vi "Periodic Tasks.vi"(8 "error in":errorcluster) -> ()   [LabVIEW 2017]
doc: "This VI runs in parallel to other tasks. It can contain as many user-defined periodic loops as you need. These can carry out PID or other sorts of timed response."
uses:
  <vilib>/Rock Robotics/Network Tables/NT Write Numeric Array.vi
  <vilib>/Rock Robotics/Network Tables/NT Write Boolean Array.vi
  Robot Global Data.vi
  <vilib>/Rock Robotics/WPI/ThirdParty/CanMotor/TalonSRX/WPI_CANTalonSRX_APIControlMode.ctl
  <vilib>/Rock Robotics/Network Tables/NT Read Number.vi
  <vilib>/Rock Robotics/Network Tables/NT Write Boolean.vi
panel:
  in  "corrector":dbl=-0.5
  in  "Slow Range":dbl=45.0
  out "Speed Closed Loop Plots 2":cluster{dbl, "Sensor Velocity":dbl}(graph)
  in  "Motor Power In":dbl=1.0
  in  "Target Range":dbl=0.5
  in  "Min Power":dbl=0.17
  out "Speed Closed Loop Plots":cluster{dbl, "Sensor Velocity":dbl}(graph)
  out "RightEncoder":dbl
  out "LeftEncoder":dbl
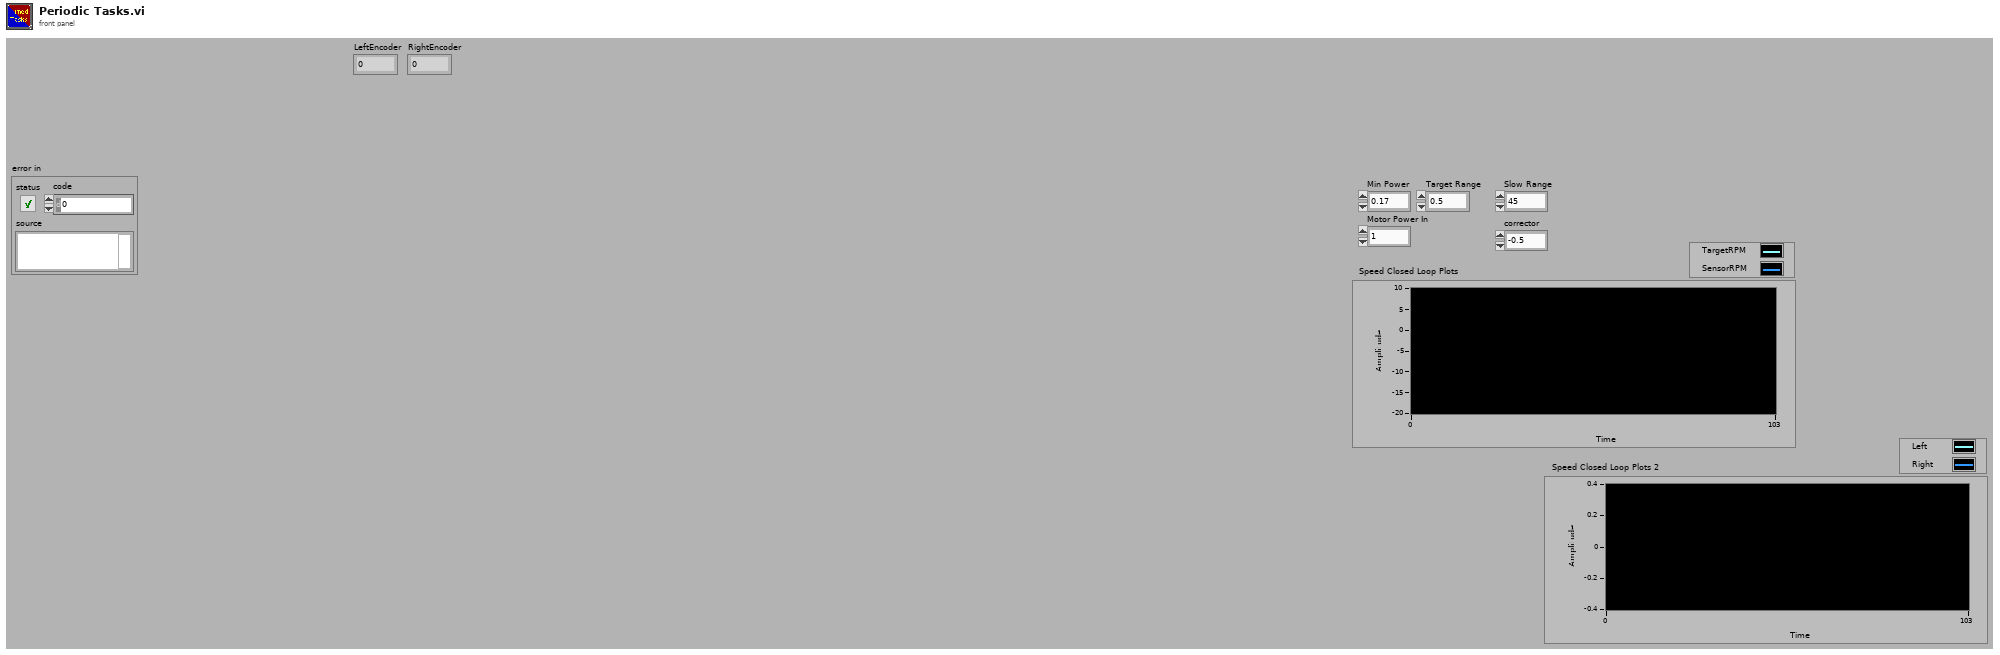
[diagram p1: front panel]
types:
  T1 = typedef "WPI_JoystickDevRef.ctl" = cluster{"Device":T2}
  T2 = typedef "WPI_JoystickDeviceEnum.ctl" = enum16{"USB 0", "USB 1", "USB 2", "USB 3", "USB 4", "USB 5"}
  T3 = cluster{"Yaw":dbl, "Roll":dbl, "Pitch":dbl, "Heading":dbl, "Fused Heading":dbl}
  T4 = typedef "WPI_CompressorDevRef.ctl" = cluster{"DevStatus":errorcluster, "Pneumatics Control Module":u8}
  T5 = enum16{"Integer", "Float", "Boolean", "Enum", "String"}
  T6 = typedef "WPI_CANTalonSRX_APIControlMode.ctl" = enum8{"Percent VBus", "Speed", "Position", "Slave", "Unchanged / Invalid", "Voltage Compensation", "Current", "Motion Profile", "Motion Magic"}
  T7 = typedef "WPI_DriverStationRobotMode2.ctl" = enum16{"Autonomous Disabled", "Autonomous Enabled", "Teleop Disabled", "Teleop Enabled", "Disconnected", "Finish", "Test Disabled", "Test Enabled", "Emergency Stopped"}
  T8 = cluster{"Buttons[0]":bool, "Buttons[1]":bool, "Buttons[2]":bool, "Buttons[3]":bool, "Buttons[4]":bool, "Buttons[5]":bool, "Buttons[6]":bool, "Buttons[7]":bool, "Buttons[8]":bool, "Buttons[9]":bool, "Buttons[10]":bool, "Buttons[11]":bool}
  T9 = cluster{"Left Motor Power":dbl, "Right Motor Power":dbl}
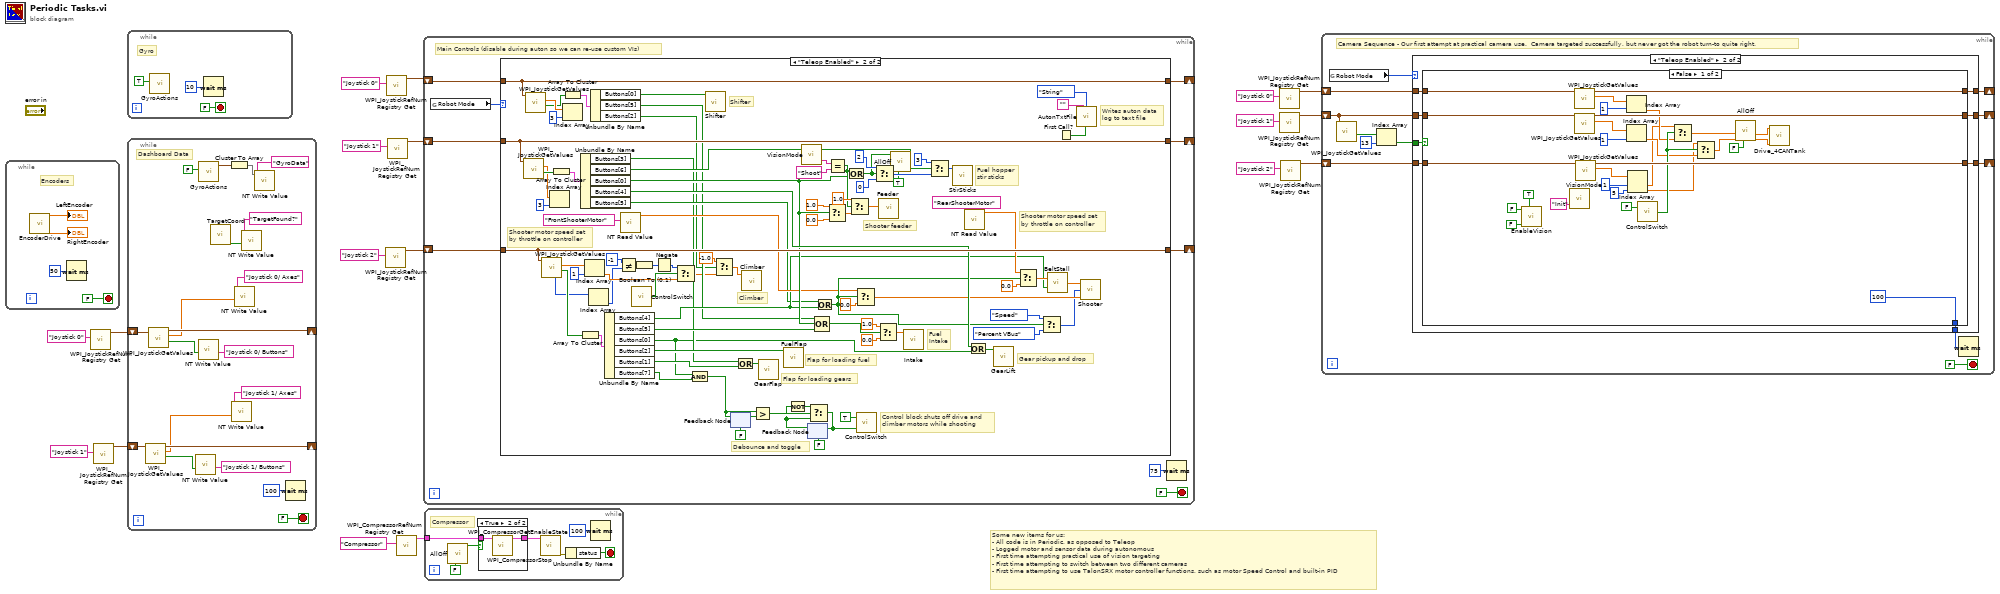
[diagram p0: block diagram]
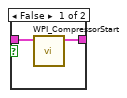
[diagram p2: hidden frame]
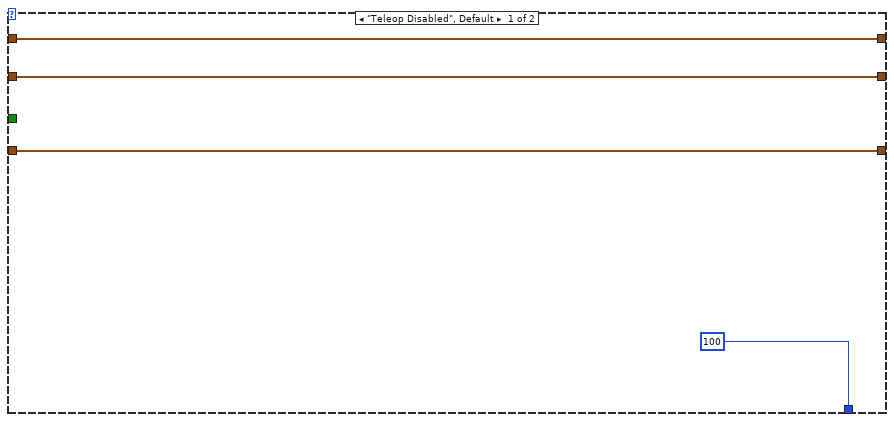
[diagram p3: hidden frame]
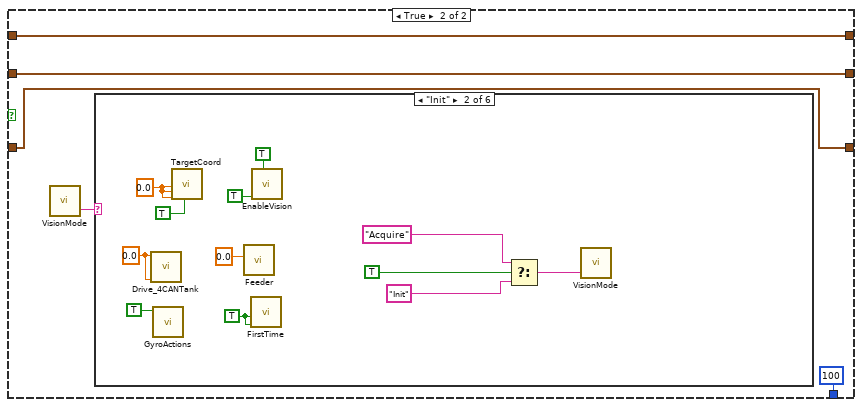
[diagram p4: hidden frame]
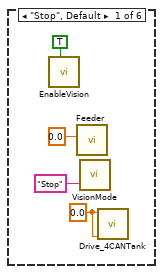
[diagram p5: hidden frame]
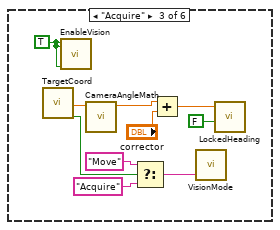
[diagram p6: hidden frame]
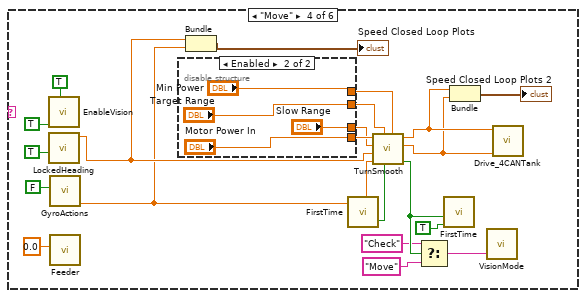
[diagram p7: hidden frame]
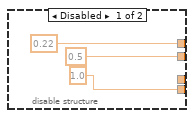
[diagram p8: hidden frame]
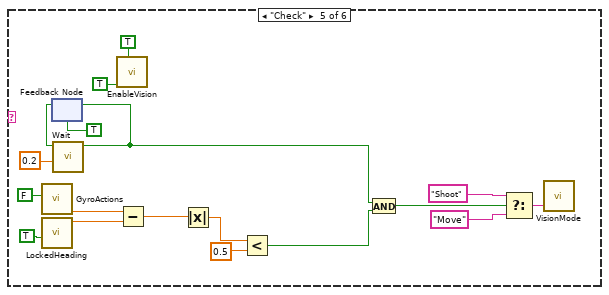
[diagram p9: hidden frame]
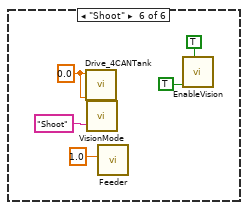
[diagram p10: hidden frame]
diagram:
  # "Some new items for us:\n- All code is in Periodic, as opposed to Teleop\n- Logged motor and sensor data during autonomous\n- First time attempting practical use of vision targeting\n- First time attempting to switch between two different cameras\n- First time attempting to use TalonSRX motor controller functions, such as motor Speed Control and built-in PID"
  n1 = while {
    stop <- FALSE stop-if-true
    # "Encoders"
    n2 = call "EncoderDrive.vi"() -> ("RightEncder"=→"RightEncoder":dbl, "LeftEncoder"=→"LeftEncoder":dbl)  [unwired: 10 in]
    n3 = Wait (ms)(milliseconds to wait=u32 50) -> ()  [unwired: 1 out]
  }
  n4 = call <vilib>:"WPI_JoystickRefNum Registry Get.vi"("refnum name"="Joystick 0") -> ("JoystickDevRef"=w16:T1)  [unwired: 9 in, 1 out]
  n5 = call <vilib>:"WPI_JoystickRefNum Registry Get.vi"("refnum name"="Joystick 1") -> ("JoystickDevRef"=w15:T1)  [unwired: 9 in, 1 out]
  n6 = while {
    stop <- FALSE stop-if-true
    # "Gyro"
    n7 = call "GyroActions.vi"("Update?"=TRUE) -> ()  [unwired: 9 in, 2 out]
    n8 = Wait (ms)(milliseconds to wait=u32 10) -> ()  [unwired: 1 out]
  }
  n9 = while {
    shift-right: [w41] -> _
    shift-left: w16 -> [w42]
    shift-right: [w33] -> _
    shift-left: w15 -> [w34]
    stop <- FALSE stop-if-true
    # "Dashboard Data"
    n10 = call <vilib>:"WPI_JoystickGetValues.vi"("JoystickDevRef"=w34) -> ("Buttons"=w37:bool[], "Axes"=w32:dbl[], "JoystickDevRef"=w33:T1)  [unwired: 6 in, 2 out]
    n11 = call <vilib>:"WPI_JoystickGetValues.vi"("JoystickDevRef"=w42) -> ("Buttons"=w39:bool[], "Axes"=w38:dbl[], "JoystickDevRef"=w41:T1)  [unwired: 6 in, 2 out]
    n12 = call-poly <vilib>:"NT Write Value.vi"("Boolean Array"=w37, "Name"="Joystick 1/ Buttons") -> ()  [unwired: 9 in, 1 out]
    n13 = call-poly <vilib>:"NT Write Value.vi"("Boolean Array"=w39, "Name"="Joystick 0/ Buttons") -> ()  [unwired: 9 in, 1 out]
    n14 = call "GyroActions.vi"("Update?"=FALSE) -> ("YRPHfH"=w29:T3)  [unwired: 9 in, 1 out]
    n15 = call "TargetCoord.vi"() -> ("Target?"=w27:bool)  [unwired: 17 in, 2 out]
    n16 = Cluster To Array(cluster=w29) -> (array=w45:dbl[])
    n17 = call-poly <vilib>:"NT Write Value.vi"("Numeric Array"=w32, "Name"="Joystick 1/ Axes") -> ()  [unwired: 9 in, 1 out]
    n18 = call-poly <vilib>:"NT Write Value.vi"("Numeric Array"=w38, "Name"="Joystick 0/ Axes") -> ()  [unwired: 9 in, 1 out]
    n19 = call-poly <vilib>:"NT Write Value.vi"("Boolean"=w27, "Name"="TargetFound?") -> ()  [unwired: 9 in, 1 out]
    n20 = call-poly <vilib>:"NT Write Value.vi"("Numeric Array"=w45, "Name"="GyroData") -> ()  [unwired: 9 in, 1 out]
    n21 = Wait (ms)(milliseconds to wait=u32 100) -> ()  [unwired: 1 out]
  }
  n22 = call <vilib>:"WPI_JoystickRefNum Registry Get.vi"("refnum name"="Joystick 2") -> ("JoystickDevRef"=w9:T1)  [unwired: 9 in, 1 out]
  n23 = call <vilib>:"WPI_JoystickRefNum Registry Get.vi"("refnum name"="Joystick 0") -> ("JoystickDevRef"=w11:T1)  [unwired: 9 in, 1 out]
  n24 = call <vilib>:"WPI_JoystickRefNum Registry Get.vi"("refnum name"="Joystick 1") -> ("JoystickDevRef"=w10:T1)  [unwired: 9 in, 1 out]
  n25 = call <vilib>:"WPI_CompressorRefNum Registry Get.vi"("refnum name"="Compressor") -> ("CompressorDevRef"=w3:T4)  [unwired: 9 in, 1 out]
  n26 = while {
    shift-right: [w47] -> _
    shift-left: w11 -> [w52]
    shift-right: [w48] -> _
    shift-left: w10 -> [w51]
    shift-right: [w49] -> _
    shift-left: w9 -> [w50]
    stop <- FALSE stop-if-true
    # "Main Controls (disable during auton so we can re-use custom VIs)"
    n27 = global read "Robot Global Data.vi" "Robot Mode"() -> (w46:T7)
    n28 = case shown="\"Teleop Enabled\"" w46 {
      tunnel: w52 -> [w57 w121]
      tunnel: w51 -> [w56 w134]
      tunnel: w50 -> [w55 w135]
      tunnel: [w55 w135] -> w49
      tunnel: [w56 w134] -> w48
      tunnel: [w57 w121] -> w47
      frame "Teleop Disabled", Default {
      }
      frame "Teleop Enabled" {
        # "Shifter"
        # "Climber"
        # "Control block shuts off drive and\nclimber motors while shooting"
        # "Shooter motor speed set\nby throttle on controller"
        # "Fuel hopper\nstir sticks"
        # "Shooter feeder"
        # "Fuel\nIntake"
        # "Gear pickup and drop"
        # "Flap for loading gears"
        # "Flap for loading fuel"
        # "Shooter motor speed set\nby throttle on controller"
        # "Debounce and toggle"
        # "Writes auton data\nlog to text file"
        n29 = call <vilib>:"WPI_JoystickGetValues.vi"("JoystickDevRef"=w134) -> ("Buttons"=w132:bool[], "Axes"=w123:dbl[])  [unwired: 6 in, 3 out]
        n30 = call <vilib>:"WPI_JoystickGetValues.vi"("JoystickDevRef"=w121) -> ("Buttons"=w114:bool[], "Axes"=w119:dbl[])  [unwired: 6 in, 3 out]
        n31 = call <vilib>:"WPI_JoystickGetValues.vi"("JoystickDevRef"=w135) -> ("Buttons"=w140:bool[], "Axes"=w143:dbl[], "POVs"=w67:i16[])  [unwired: 6 in, 2 out]
        n32 = Index Array(array=w123, index=3) -> ()  [unwired: 1 out]
        n33 = Array To Cluster(array=w132) -> (cluster=w133:T8)
        n34 = Array To Cluster(array=w114) -> (cluster=w115:T8)
        n35 = Index Array(array=w119, index=3) -> ()  [unwired: 1 out]
        n36 = Array To Cluster(array=w140) -> (cluster=w141:T8)
        n37 = Unbundle By Name(w133) -> ("Buttons[3]"=w79:bool, "Buttons[6]"=w85:bool, "Buttons[0]"=w107:bool, "Buttons[4]"=w124:bool, "Buttons[5]"=w86:bool)
        n38 = Index Array(array=w143, index=1) -> (element=w64:dbl)
        n39 = Index Array(array=w67) -> (element=w63:i16)  [unwired: 1 in]
        n40 = Unbundle By Name(w115) -> ("Buttons[0]"=w113:bool, "Buttons[5]"=w84:bool, "Buttons[2]"=w82:bool)
        n41 = Unbundle By Name(w141) -> ("Buttons[4]"=w87:bool, "Buttons[5]"=w97:bool, "Buttons[0]"=w60:bool, "Buttons[2]"=w136:bool, "Buttons[1]"=w77:bool, "Buttons[7]"=w78:bool)
        n42 = Not Equal?(x=i16 -1, y=w63) -> (x != y?=w61:bool)
        n43 = call-poly <vilib>:"NT Read Value.vi"("Name"="FrontShooterMotor") -> ("Numeric"=w93:dbl)  [unwired: 9 in, 1 out]
        n44 = call "ControlSwitch.vi"() -> ("ControlsSwitchOut"=w65:bool)  [unwired: 2 in]
        n45 = Boolean To (0,1)(Boolean=w61) -> (0, 1=w59:i16)
        n46 = Negate(x=w59) -> (-x=w58:i16)
        n47 = Select(t=w58, s=w65, f=w64) -> (s? t:f=w66:dbl)
        n48 = And(x=w60, y=w78) -> (x .and. y?=w70:bool)
        n49 = call "Shifter.vi"("Shift"=w113) -> ()  [unwired: 11 in]
        n50 = Select(t=-1.0, s=w82, f=w66) -> (s? t:f=w83:dbl)
        n51 = feedback #1(FALSE ("Fuel Flap")) -> (w75:bool)
        n52 = feedback-in #1(w70) -> ()
        n53 = Or(x=w79, y=w77) -> (x .or. y?=w80:bool)
        n54 = call "Climber.vi"("Power"=w83) -> ()  [unwired: 11 in]
        n55 = Greater?(x=w70, y=w75) -> (0:w74:bool)
        n56 = call "GearFlap.vi"("Gear Flap"=w80) -> ()  [unwired: 11 in]
        n57 = call "FuelFlap.vi"("Fuel Flap"=w136) -> ()  [unwired: 11 in]
        n58 = call "VisionMode.vi"() -> ("ModeOut"=w129:string)  [unwired: 3 in]
        n59 = feedback #2(FALSE) -> (w72:bool)
        n60 = Not(x=w72) -> (.not. x?=w73:bool)
        n61 = Select(t=w73, s=w74, f=w72) -> (s? t:f=w68:bool)
        n62 = feedback-in #2(w68) -> ()
        n63 = Compound Arithmetic op=OR(w84, w107, w97) -> (w112:bool)
        n64 = Or(x=w86, y=w87) -> (x .or. y?=w98:bool)
        n65 = Select(t=1.0, s=w107, f=0.0) -> (s? t:f=w127:dbl)
        n66 = Equal?(x=w129, y="Shoot" ("ModeIn")) -> (x = y?=w109:bool)
        n67 = Or(x=w109, y=w107) -> (x .or. y?=w106:bool)
        n68 = Select(t=1.0, s=w109, f=w127) -> (s? t:f=w108:dbl)
        n69 = Select(t=w93, s=w98, f=0.0) -> (s? t:f=w105:dbl)
        n70 = call "ControlSwitch.vi"("ControlsSwitch"=w68, "Update"=TRUE) -> ()  [unwired: 1 out]
        n71 = Select(t=i16 2, s=w106, f=i16 0) -> (s? t:f=w118:i16)
        n72 = Select(t=1.0, s=w112, f=0.0) -> (s? t:f=w137:dbl)
        n73 = call "Feeder.vi"("Power"=w108) -> ()  [unwired: 11 in]
        n74 = call "AllOff.vi"("Update?"=TRUE, "ButtonIn"=w106) -> ()  [unwired: 7 in, 3 out]
        n75 = call "Intake.vi"("Power"=w137) -> ()  [unwired: 11 in]
        n76 = Select(t=i16 3, s=w85, f=w118) -> (s? t:f=w117:i16)
        n77 = call "StirSticks.vi"("RelayValue"=w117) -> ()  [unwired: 11 in]
        n78 = call-poly <vilib>:"NT Read Value.vi"("Name"="RearShooterMotor") -> ("Numeric"=w94:dbl)  [unwired: 9 in, 1 out]
        n79 = Or(x=w124, y=w60) -> (x .or. y?=w125:bool)
        n80 = call "GearLift.vi"("Gear Up"=w125) -> ()  [unwired: 11 in]
        n81 = Select(t=w94, s=w98, f=0.0) -> (s? t:f=w90:dbl)
        n82 = Select(t=WPI_CANTalonSRX_APIControlMode."Speed" ("Control Mode"), s=w98, f=WPI_CANTalonSRX_APIControlMode."Percent VBus" ("Control Mode")) -> (s? t:f=w101:T6)
        n83 = call "BeltStall.vi"("Boolean"=w87, "BeltSpeed"=w90) -> ("BeltSpeedOut"=w89:dbl)
        n84 = First Call?() -> (First Call?: T/F=w92:bool)
        n85 = call "AutonTxtFile.vi"("dataName"="", "mode"=T5."String", "writeToFile?"=w92) -> ()  [unwired: 11 in, 2 out]
        n86 = call "Shooter.vi"("FrontMotorIn"=w105, "Control Mode"=w101, "RearMotorIn"=w89) -> ()  [unwired: 1 in]
      }
    }
    n87 = Wait (ms)(milliseconds to wait=u32 75) -> ()  [unwired: 1 out]
  }
  n88 = while {
    tunnel: w3 -> [w148]
    stop <- w149 stop-if-true
    # "Compressor"
    n89 = call "AllOff.vi"("Update?"=FALSE) -> ("Compressor"=w145:bool)  [unwired: 8 in, 2 out]
    n90 = case shown="True" w145 {
      tunnel: w148 -> [w152 w154]
      tunnel: [w151 w153] -> w147
      frame False {
        n91 = call <vilib>:"WPI_CompressorStart.vi"("CompressorDevRef"=w152) -> ("CompressorDevRef"=w151:T4)  [unwired: 9 in, 1 out]
      }
      frame True {
        n92 = call <vilib>:"WPI_CompressorStop.vi"("CompressorDevRef"=w154) -> ("CompressorDevRef"=w153:T4)  [unwired: 9 in, 1 out]
      }
    }
    n93 = call <vilib>:"WPI_CompressorGetEnableState.vi"("CompressorDevRef"=w147) -> ("error out"=w146:errorcluster)  [unwired: 1 in, 9 out]
    n94 = Unbundle By Name(w146) -> ("status"=w149:bool)
    n95 = Wait (ms)(milliseconds to wait=u32 100) -> ()  [unwired: 1 out]
  }
  n96 = call <vilib>:"WPI_JoystickRefNum Registry Get.vi"("refnum name"="Joystick 0") -> ("JoystickDevRef"=w8:T1)  [unwired: 9 in, 1 out]
  n97 = call <vilib>:"WPI_JoystickRefNum Registry Get.vi"("refnum name"="Joystick 1") -> ("JoystickDevRef"=w7:T1)  [unwired: 9 in, 1 out]
  n98 = call <vilib>:"WPI_JoystickRefNum Registry Get.vi"("refnum name"="Joystick 2") -> ("JoystickDevRef"=w1:T1)  [unwired: 9 in, 1 out]
  n99 = while {
    shift-right: [w163] -> _
    shift-left: w8 -> [w164]
    shift-right: [w162] -> _
    shift-left: w7 -> [w160]
    shift-right: [w155] -> _
    shift-left: w1 -> [w156]
    stop <- FALSE stop-if-true
    # "Camera Sequence - Our first attempt at practical camera use.  Camera targeted successfully, but never got the robot turn-to quite right."
    n100 = global read "Robot Global Data.vi" "Robot Mode"() -> (w165:T7)
    n101 = call <vilib>:"WPI_JoystickGetValues.vi"("JoystickDevRef"=w160) -> ("Buttons"=w159:bool[])  [unwired: 6 in, 4 out]
    n102 = Index Array(array=w159, index=13) -> (element=w157:bool)
    n103 = case shown="\"Teleop Enabled\"" w165 {
      tunnel: w164 -> [w170 w178]
      tunnel: w160 -> [w169 w177]
      tunnel: [w170 w176] -> w163
      tunnel: [w169 w175] -> w162
      tunnel: [100 w174] -> w161
      tunnel: w157 -> [_ w173]
      tunnel: w156 -> [w167 w172]
      tunnel: [w167 w171] -> w155
      frame "Teleop Disabled", Default {
      }
      frame "Teleop Enabled" {
        n104 = case shown="False" w173 {
          tunnel: w178 -> [w207 w212]
          tunnel: w177 -> [w206 w211]
          tunnel: [w205 w212] -> w176
          tunnel: [w204 w211] -> w175
          tunnel: [100 100] -> w174
          tunnel: w172 -> [w189 w208]
          tunnel: [w188 w208] -> w171
          frame False {
            n105 = call "EnableVision.vi"("Update"=TRUE, "VisionButton"=FALSE, "EnableVision"=FALSE) -> ()  [unwired: 7 in, 2 out]
            n106 = call "VisionMode.vi"("ModeIn"="Init") -> ()  [unwired: 2 in, 1 out]
            n107 = call <vilib>:"WPI_JoystickGetValues.vi"("JoystickDevRef"=w207) -> ("Axes"=w199:dbl[], "JoystickDevRef"=w205:T1)  [unwired: 6 in, 3 out]
            n108 = call <vilib>:"WPI_JoystickGetValues.vi"("JoystickDevRef"=w206) -> ("Axes"=w198:dbl[], "JoystickDevRef"=w204:T1)  [unwired: 6 in, 3 out]
            n109 = call <vilib>:"WPI_JoystickGetValues.vi"("JoystickDevRef"=w189) -> ("Axes"=w187:dbl[], "JoystickDevRef"=w188:T1)  [unwired: 6 in, 3 out]
            n110 = Index Array(array=w199, index=1) -> (element=w180:dbl)
            n111 = Index Array(array=w198, index=1) -> (element=w182:dbl)
            n112 = Index Array(array=w187, index #1=1 ("index"), index #2=5 ("index")) -> (element #1=w179:dbl, element #2=w181:dbl)
            n113 = call "ControlSwitch.vi"("Update"=FALSE) -> ("ControlsSwitchOut"=w184:bool)  [unwired: 1 in]
            n114 = Select(t=w179, s=w184, f=w180) -> (s? t:f=w185:dbl)
            n115 = Select(t=w181, s=w184, f=w182) -> (s? t:f=w183:dbl)
            n116 = call "AllOff.vi"("Update?"=FALSE, "RightIn"=w183, "LeftIn"=w185) -> ("RightOut"=w195:dbl, "LeftOut"=w194:dbl)  [unwired: 6 in, 1 out]
            n117 = call "Drive_4CANTank.vi"("RightMotor"=w195, "LeftMotor"=w194) -> ()  [unwired: 10 in]
          }
          frame True {
            n118 = call "VisionMode.vi"() -> ("ModeOut"=w209:string)  [unwired: 3 in]
            n119 = case shown="\"Init\"" w209 {
              frame "Stop", Default {
                w216 = 0.0 ("Motor Power Out")
                n120 = call "EnableVision.vi"("Update"=TRUE) -> ()  [unwired: 9 in, 2 out]
                n121 = call "Feeder.vi"("Power"=0.0) -> ()  [unwired: 11 in]
                n122 = call "VisionMode.vi"("ModeIn"="Stop") -> ()  [unwired: 2 in, 1 out]
                n123 = call "Drive_4CANTank.vi"("RightMotor"=w216, "LeftMotor"=w216) -> ()  [unwired: 10 in]
              }
              frame "Init" {
                w224 = 0.0 ("CenterXIn")
                w227 = 0.0 ("Motor Power Out")
                w225 = TRUE ("Input")
                n124 = call "Drive_4CANTank.vi"("RightMotor"=w227, "LeftMotor"=w227) -> ()  [unwired: 10 in]
                n125 = call "GyroActions.vi"("Zero"=TRUE) -> ()  [unwired: 9 in, 2 out]
                n126 = call "TargetCoord.vi"("CenterXIn"=w224, "CenterYIn"=w224, "ScoreIn"=w224, "Update?"=TRUE) -> ()  [unwired: 13 in, 3 out]
                n127 = call "Feeder.vi"("Power"=0.0) -> ()  [unwired: 11 in]
                n128 = call "FirstTime"("Update?"=w225, "Input"=w225) -> ()  [unwired: 3 in, 1 out]
                n129 = call "EnableVision.vi"("Update"=TRUE, "VisionButton"=TRUE) -> ()  [unwired: 8 in, 2 out]
                n130 = Select(t="Acquire" ("ModeIn"), s=TRUE, f="Init") -> (s? t:f=w220:string)
                n131 = call "VisionMode.vi"("ModeIn"=w220) -> ()  [unwired: 2 in, 1 out]
              }
              frame "Acquire" {
                w232 = TRUE ("EnableVision")
                n132 = call "TargetCoord.vi"() -> ("CenterXOut"=w237:dbl, "Target?"=w236:bool)  [unwired: 17 in, 1 out]
                n133 = call "EnableVision.vi"("Update"=w232, "VisionButton"=w232, "EnableVision"=w232) -> ()  [unwired: 7 in, 2 out]
                n134 = call "CameraAngleMath.vi"("TargetXCenter"=w237) -> ("TargetAngle"=w230:dbl)  [unwired: 10 in]
                n135 = Select(t="Move" ("ModeIn"), s=w236, f="Acquire" ("ModeIn")) -> (s? t:f=w235:string)
                n136 = Add(x=w230, y="corrector") -> (x+y=w231:dbl)
                n137 = call "VisionMode.vi"("ModeIn"=w235) -> ()  [unwired: 2 in, 1 out]
                n138 = call "LockedHeading.vi"("LockHeading"=FALSE, "Heading In"=w231) -> ()  [unwired: 9 in, 1 out]
              }
              frame "Move" {
                n139 = call "EnableVision.vi"("Update"=TRUE ("EnableVision"), "VisionButton"=TRUE) -> ()  [unwired: 8 in, 2 out]
                n140 = call "LockedHeading.vi"("LockHeading"=TRUE) -> ("LockedHeading"=w258:dbl)  [unwired: 10 in]
                n141 = call "GyroActions.vi"("Update?"=FALSE) -> ("Yaw"=w246:dbl)  [unwired: 9 in, 1 out]
                n142 = call "Feeder.vi"("Power"=0.0) -> ()  [unwired: 11 in]
                n143 = disable-structure shown="Enabled" {
                  disable-tunnel: [0.5 ("Target Range") "Target Range"] -> w243
                  disable-tunnel: [0.22 ("Min Power") "Min Power"] -> w242
                  disable-tunnel: [1.0 ("Motor Power In") "Motor Power In"] -> w241
                  disable-tunnel: [_ "Slow Range"] -> w239
                  frame Disabled {
                  }
                  frame Enabled {
                  }
                }
                n144 = Bundle("LockedHeading"=w258, "Yaw"=w246) -> (→"Speed Closed Loop Plots":cluster{"LockedHeading":dbl, "Yaw":dbl})  [unwired: 1 in]
                n145 = call "FirstTime"() -> ("Output"=w244:bool)  [unwired: 5 in]
                n146 = call "TurnSmooth.vi"("Min Power"=w242, "First Time?"=w244, "Target Range"=w243, "Current Position"=w246, "Target Position"=w258, "Slow Range"=w239, "Motor Power In"=w241) -> ("Done"=w257:bool, "Right Motor Power"=w254:dbl, "Left Motor Power"=w255:dbl)  [unwired: 2 in]
                n147 = Select(t="Check", s=w257, f="Move") -> (s? t:f=w251:string)
                n148 = call "FirstTime"("Update?"=TRUE, "Input"=w257) -> ()  [unwired: 3 in, 1 out]
                n149 = Bundle("Left Motor Power"=w255, "Right Motor Power"=w254) -> (→"Speed Closed Loop Plots 2":T9)  [unwired: 1 in]
                n150 = call "VisionMode.vi"("ModeIn"=w251) -> ()  [unwired: 2 in, 1 out]
                n151 = call "Drive_4CANTank.vi"("RightMotor"=w254, "LeftMotor"=w255) -> ()  [unwired: 10 in]
              }
              frame "Check" {
                n152 = call "GyroActions.vi"("Update?"=FALSE) -> ("Yaw"=w279:dbl)  [unwired: 9 in, 1 out]
                n153 = call "LockedHeading.vi"("LockHeading"=TRUE) -> ("LockedHeading"=w280:dbl)  [unwired: 10 in]
                n154 = feedback #3(TRUE ("Completed")) -> (w275:bool)
                n155 = call "Wait.vi"("Target Time (s)"=0.2 ("Target Time"), "First Time?"=w275) -> ("Completed"=w270:bool)  [unwired: 9 in]
                n156 = feedback-in #3(w270) -> ()
                n157 = call "EnableVision.vi"("Update"=TRUE, "VisionButton"=TRUE) -> ()  [unwired: 8 in, 2 out]
                n158 = Subtract(x=w279, y=w280) -> (x-y=w278:dbl)
                n159 = Absolute Value(x=w278) -> (abs(x)=w277:dbl)
                n160 = Less?(x=w277, y=0.5) -> (x < y?=w271:bool)
                n161 = And(x=w270, y=w271) -> (x .and. y?=w272:bool)
                n162 = Select(t="Shoot", s=w272, f="Move") -> (s? t:f=w282:string)
                n163 = call "VisionMode.vi"("ModeIn"=w282) -> ()  [unwired: 2 in, 1 out]
              }
              frame "Shoot" {
                w289 = 0.0 ("Motor Power Out")
                n164 = call "Drive_4CANTank.vi"("RightMotor"=w289, "LeftMotor"=w289) -> ()  [unwired: 10 in]
                n165 = call "VisionMode.vi"("ModeIn"="Shoot") -> ()  [unwired: 2 in, 1 out]
                n166 = call "Feeder.vi"("Power"=1.0) -> ()  [unwired: 11 in]
                n167 = call "EnableVision.vi"("Update"=TRUE, "VisionButton"=TRUE) -> ()  [unwired: 8 in, 2 out]
              }
            }
          }
        }
      }
    }
    n168 = Wait (ms)(milliseconds to wait=w161) -> ()  [unwired: 1 out]
  }
